vi "CANOpen EDS string to value.vi"(9 "DefaultValue":string, 10 "DataType":T2 items=[""=0, "BOOLEAN"=1, "INTEGER8"=2, "INTEGER16"=3, "INTEGER32"=4, "UNSIGNED8"=5, "UNSIGNED16"=6, "UNSIGNED32"=7, "REAL32"=8, "VISIBLE_STRING"=9, "OCTET_STRING"=10, "UNICODE_STRING"=11, "TIME_OF_DAY"=12, "TIME_DIFFERENCE"=13, "DOMAIN"=15, "INTEGER24"=16, "REAL64"=17, "INTEGER40"=18, "INTEGER48"=19, "INTEGER56"=20, "INTEGER64"=21, "UNSIGNED24"=22, "UNSIGNED40"=24, "UNSIGNED48"=25, "UNSIGNED56"=26, "UNSIGNED64"=27]) -> (1 "Disabled":T1(ring), 2 "Block Data":u8[](array[numeric]) format="%.0x", 3 "Translated value":i64, 4 "Disabled float":T1(ring), 5 "Translated value float":dbl)   [LabVIEW 2013, in "CANOpen Addon Custom Device.lvlib"]
uses:
  CANOpen Addon Custom Device.lvlib
  EDS/control/Data Type.ctl
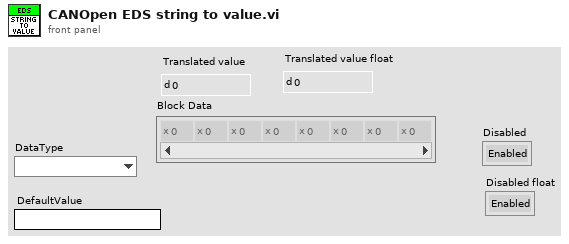
[diagram p1: front panel]
types:
  T1 = enum8{"Enabled", "Disabled", "Disabled and Grayed Out"}
  T2 = typedef "Data Type.ctl" = u16
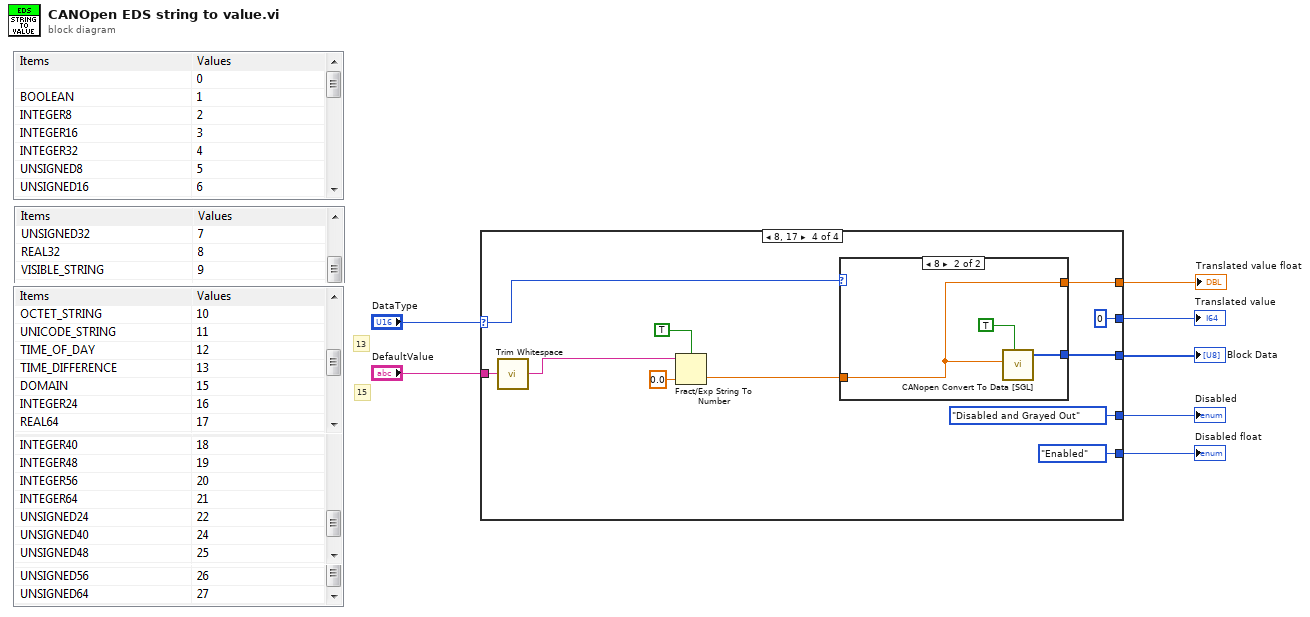
[diagram p0: block diagram]
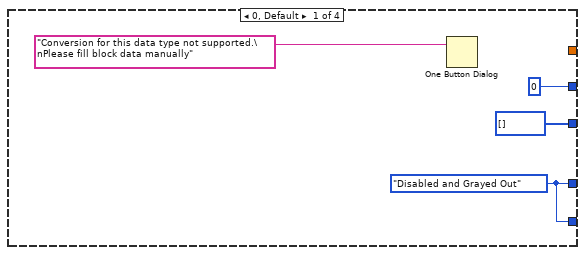
[diagram p2: hidden frame]
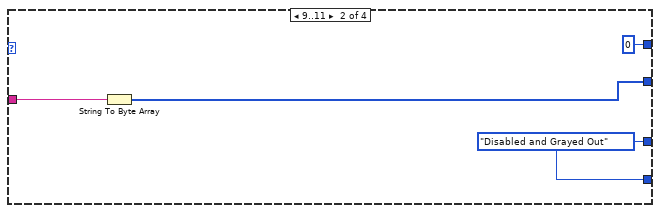
[diagram p3: hidden frame]
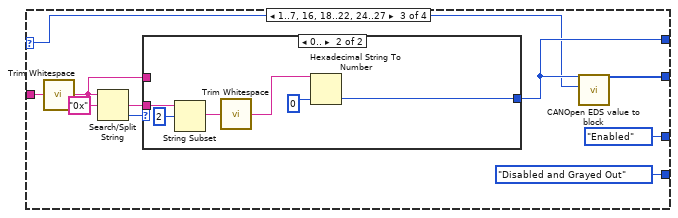
[diagram p4: hidden frame]
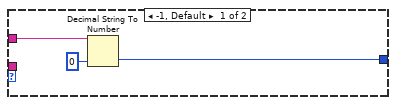
[diagram p5: hidden frame]
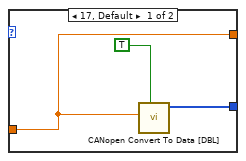
[diagram p6: hidden frame]
diagram:
  # "15"
  # "13"
  n1 = case shown="8, 17" "DataType" {
    selector: "DataType" -> [_ _ w17 w42]
    tunnel: [i64 0 ("Translated value") i64 0 ("Translated value") w19 i64 0 ("Translated value")] -> w3
    tunnel: [w8 w12 T1."Enabled" ("Disabled") T1."Disabled and Grayed Out" ("Disabled")] -> w6
    tunnel: [u8[] [] ("Block Data") w14 w18 w41] -> w5
    tunnel: "DefaultValue" -> [_ w15 w25 w45]
    tunnel: [w8 w12 T1."Disabled and Grayed Out" ("Disabled") T1."Enabled" ("Disabled")] -> w2
    tunnel: [_ _ _ w37] -> w1
    frame 0, Default {
      w8 = T1."Disabled and Grayed Out" ("Disabled")
      n2 = One Button Dialog(message="Conversion for this data type not supported.\nPlease fill block data manually") -> ()  [unwired: 1 in, 1 out]
    }
    frame 9..11 {
      w12 = T1."Disabled and Grayed Out" ("Disabled")
      n3 = String To Byte Array(string=w15) -> (unsigned byte array=w14:u8[])
    }
    frame 1..7, 16, 18..22, 24..27 {
      n4 = call <vilib>:"Trim Whitespace.vi"("string"=w25) -> ("trimmed string"=w22:string)  [unwired: 1 in]
      n5 = Search/Split String(string=w22, search string/char (-)="0x") -> (match + rest of string=w21:string, offset of match=w23:i32)  [unwired: 1 in, 1 out]
      n6 = case shown="0.." w23 {
        tunnel: w22 -> [w27 _]
        tunnel: w21 -> [_ w34]
        tunnel: [w26 w30] -> w19
        frame -1, Default {
          n7 = Decimal String To Number(string=w27, default (0L)=i64 0 ("Translated value")) -> (number=w26:i64)  [unwired: 1 in, 1 out]
        }
        frame 0.. {
          n8 = String Subset(string=w34, offset (0)=2) -> (substring=w32:string)  [unwired: 1 in]
          n9 = call <vilib>:"Trim Whitespace.vi"("string"=w32) -> ("trimmed string"=w29:string)  [unwired: 1 in]
          n10 = Hexadecimal String To Number(string=w29, default (0uL)=i64 0 ("Translated value")) -> (number=w30:i64)  [unwired: 1 in, 1 out]
        }
      }
      n11 = call "CANOpen EDS value to block.vi"("DataType"=w17, "Translated value"=w19) -> ("Block Data"=w18:u8[])  [unwired: 9 in]
    }
    frame 8, 17 {
      n12 = call <vilib>:"Trim Whitespace.vi"("string"=w45) -> ("trimmed string"=w44:string)  [unwired: 1 in]
      n13 = Fract/Exp String To Number(use system decimal point (T)=TRUE, string=w44, default (0 dbl)=0.0 ("Translated value")) -> (number=w40:dbl)  [unwired: 1 in, 1 out]
      n14 = case shown="8" w42 {
        tunnel: [w47 w50] -> w41
        tunnel: w40 -> [w46 w49]
        tunnel: [w46 w49] -> w37
        frame 17, Default {
          n15 = call <vilib>:"CANopen Convert To Data [DBL].vi"("trim"=TRUE, "8-byte double"=w46) -> ("CANopen data out"=w47:u8[])  [unwired: 8 in, 1 out]
        }
        frame 8 {
          n16 = call <vilib>:"CANopen Convert To Data [SGL].vi"("trim"=TRUE, "4-byte single"=w49) -> ("CANopen data out"=w50:u8[])  [unwired: 8 in, 1 out]
        }
      }
    }
  }
  "Block Data" <- w5
  "Disabled" <- w6
  "Translated value" <- w3
  "Disabled float" <- w2
  "Translated value float" <- w1
